vi "dataUpload.vi"(0 "upload":bool, 1 "uploadpath":path, 3 "status msg ref":refnum<vi>, 4 "sn":string, 5 "错误输入（无错误）":errorcluster, 6 "pn":string, 7 "DBSet":T1, 8 "xmlPath":path, 14 "result":string) -> (19 "错误输出":errorcluster)   [LabVIEW 2011]
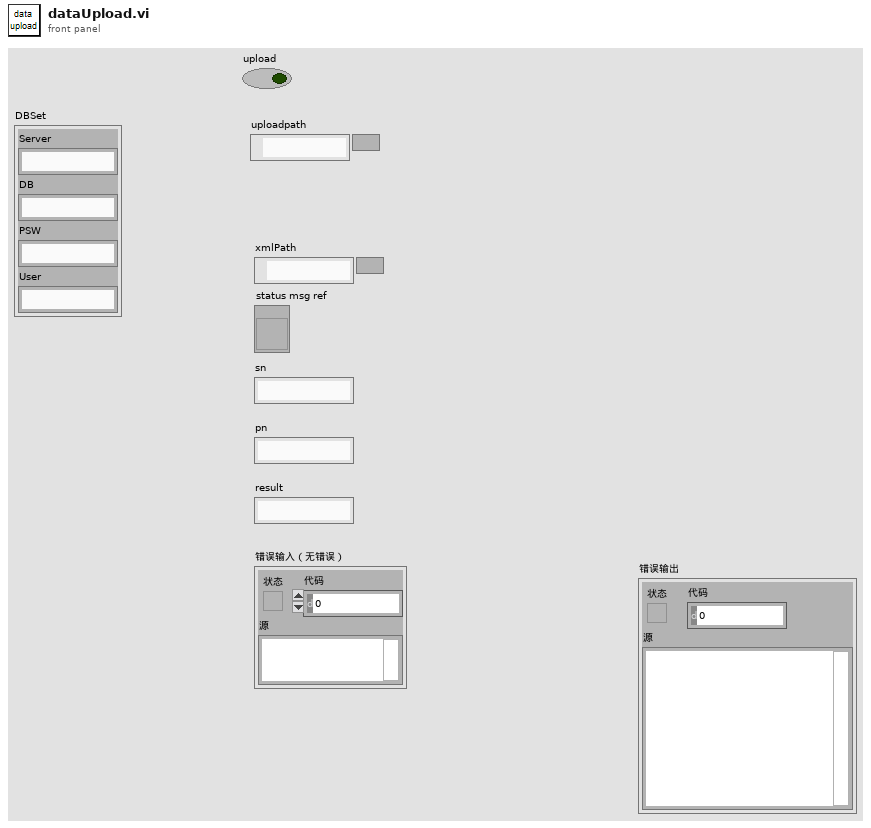
[diagram p1: front panel]
types:
  T1 = cluster{"Server":string, "DB":string, "PSW":string, "User":string}
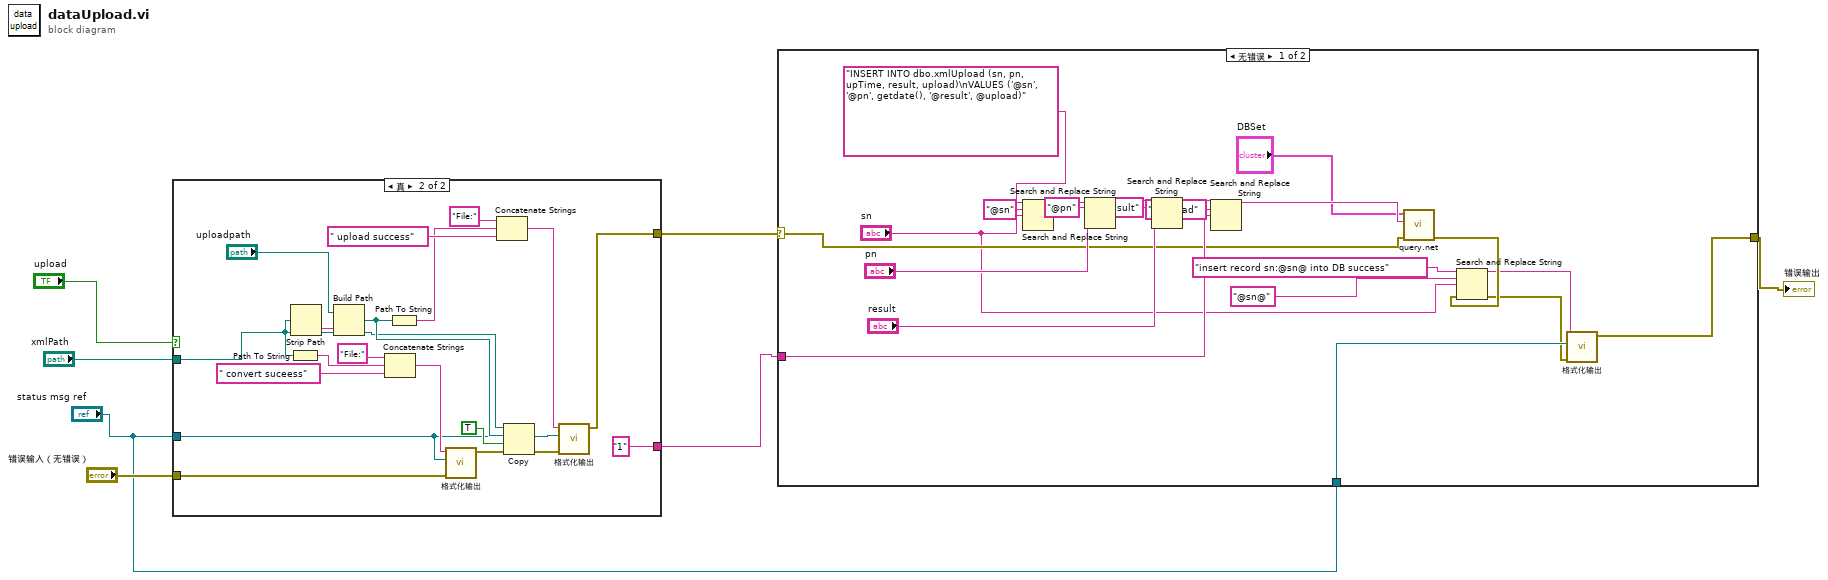
[diagram p0: block diagram]
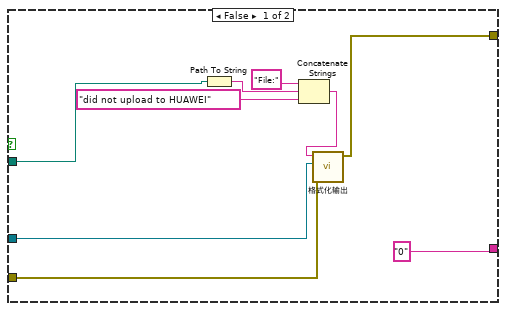
[diagram p2: hidden frame]
diagram:
  n1 = case shown="真" "upload" {
    tunnel: [w9 w22] -> w7
    tunnel: "错误输入（无错误）" -> [w10 w21]
    tunnel: "status msg ref" -> [w11 w20]
    tunnel: "xmlPath" -> [w13 w19]
    tunnel: ["0" "1"] -> w2
    frame False {
      n2 = Path To String(path=w13) -> (string=w15:string)
      n3 = Concatenate Strings("File:" ("字符串"), w15, "did not upload to HUAWEI" ("字符串")) -> (w12:string)
      n4 = call "格式化输出.vi"("错误输入（无错误）"=w10, "字符串引用"=w11, "字符串"=w12) -> ("错误输出"=w9:errorcluster)  [unwired: 8 in]
    }
    frame True {
      n5 = Path To String(path=w19) -> (string=w34:string)
      n6 = Strip Path(path=w19) -> (name=w30:string)  [unwired: 1 out]
      n7 = Build Path(base path="uploadpath", name or relative path=w30) -> (appended path=w24:path)
      n8 = Concatenate Strings("File:" ("字符串"), w34, " convert suceess" ("字符串")) -> (w32:string)
      n9 = Path To String(path=w24) -> (string=w23:string)
      n10 = call "格式化输出.vi"("错误输入（无错误）"=w21, "字符串引用"=w20, "字符串"=w32) -> ("错误输出"=w29:errorcluster)  [unwired: 8 in]
      n11 = Concatenate Strings("File:" ("字符串"), w23, " upload success") -> (w25:string)
      n12 = Copy(8:w29, 9:TRUE ("覆盖(F)"), 10:w24, 11:w19) -> (0:w26:errorcluster)  [unwired: 1 in, 2 out]
      n13 = call "格式化输出.vi"("错误输入（无错误）"=w26, "字符串引用"=w20, "字符串"=w25) -> ("错误输出"=w22:errorcluster)  [unwired: 8 in]
    }
  }
  n14 = case shown="无错误" w7 {
    selector: w7 -> [w44 w58]
    tunnel: w2 -> [w47 _]
    tunnel: [w37 w58] -> w6
    tunnel: "status msg ref" -> [w43 _]
    frame No Error {
      n15 = Search and Replace String(input string="INSERT INTO dbo.xmlUpload (sn, pn, upTime, result, upload)\nVALUES ('@sn', '@pn', getdate(), '@result', @upload)", search string="@sn" ("搜索字符串"), replace string="sn") -> (result string=w50:string)  [unwired: 5 in, 3 out]
      n16 = Search and Replace String(input string=w50, search string="@pn" ("搜索字符串"), replace string="pn") -> (result string=w53:string)  [unwired: 5 in, 3 out]
      n17 = Search and Replace String(input string=w53, search string="@result" ("搜索字符串"), replace string="result") -> (result string=w56:string)  [unwired: 5 in, 3 out]
      n18 = Search and Replace String(input string=w56, search string="@upload" ("搜索字符串"), replace string=w47) -> (result string=w46:string)  [unwired: 5 in, 3 out]
      n19 = call "query.net.vi"("错误输入（无错误）"=w44, "Sql"=w46, "DBSet"="DBSet") -> ("错误输出"=w39:errorcluster)  [unwired: 7 in, 1 out]
      n20 = Search and Replace String(input string="insert record sn:@sn@ into DB success", search string="@sn@" ("搜索字符串"), replace string="sn", error in=w39) -> (result string=w36:string, error out=w38:errorcluster)  [unwired: 4 in, 2 out]
      n21 = call "格式化输出.vi"("错误输入（无错误）"=w38, "字符串引用"=w43, "字符串"=w36) -> ("错误输出"=w37:errorcluster)  [unwired: 8 in]
    }
    frame Error {
    }
  }
  "错误输出" <- w6
